vi "HFRR ADV v01.vi"() -> ()   [LabVIEW 2023] (continued)
                  n214 = VISA Read(VISA resource name=w509, byte count=w500, error in (no error)=w508) -> (VISA resource name out=w506:refnum<visa-resource-name>, read buffer=w498:string, error out=w507:errorcluster)  [unwired: 1 out]
                  n215 = Concatenate Strings(w499, w498) -> (w497:string)
                }
                "UnoRead" <- w449
                n216 = while {
                  shift-right: [w483] -> w460
                  shift-left: w449 -> [w489]
                  tunnel: [w482] -> w456 mode=indexing
                  tunnel: [w484] -> _
                  i -> [w484]
                  stop <- w486 stop-if-true
                  n217 = Match Pattern(string=w489, regular expression="*") -> (after substring=w487:string)  [unwired: 1 in, 3 out]
                  n218 = Match Pattern(string=w487, regular expression="&") -> (before substring=w482:string, after substring=w483:string, offset past match=w485:i32)  [unwired: 1 in, 1 out]
                  n219 = Less Than 0?(x=w485) -> (x < 0?=w486:bool)
                }
                n220 = local write "Residual Uno"(w460) -> ()
                n221 = Array Size(array=w456) -> (size(s)=w457:i32)
                n222 = Decrement(x=w457) -> (x-1=w459:i32)
                n223 = Delete From Array(array=w456, length=1, index=w459) -> (array with subset deleted=w454:string[])  [unwired: 1 out]
                n224 = Array Size(array=w454) -> (size(s)=w453:i32)
                n225 = Decrement(x=w453) -> (x-1=w452:i32)
                n226 = while {
                  tunnel: [w481] -> w465 mode=indexing
                  tunnel: [w480] -> w464 mode=indexing
                  tunnel: w454 -> [w474] mode=indexing
                  tunnel: w452 -> [w473]
                  tunnel: [w471] -> _
                  i -> [w471]
                  stop <- w472 stop-if-true
                  w475 = 0 ("length (rest)")
                  w477 = ";" ("regular expression")
                  n227 = Match Pattern(string=w474, regular expression=w477) -> (before substring=w479:string, after substring=w478:string)  [unwired: 1 in, 2 out]
                  n228 = Match Pattern(string=w478, regular expression=w477) -> (before substring=w476:string)  [unwired: 1 in, 3 out]
                  n229 = Less Or Equal?(x=w473, y=w471) -> (x <= y?=w472:bool)
                  n230 = Decimal String To Number(string=w479, default (0L)=w475) -> (number=w481:i32)  [unwired: 1 in, 1 out]
                  n231 = Decimal String To Number(string=w476, default (0L)=w475) -> (number=w480:i32)  [unwired: 1 in, 1 out]
                }
                n232 = Bundle(w465, w464) -> (w455:cluster{i32[], i32[]})  [unwired: 1 in]
                n233 = case shown="0, Default" "ADC Res" {
                  tunnel: [w492 w494] -> w448
                  frame 0, Default {
                    n234 = Divide(x=65535 ("length (rest)"), y=2 ("length (rest)")) -> (x/y=w492:dbl)
                  }
                  frame 1 {
                    n235 = Divide(x=16777216 ("length (rest)"), y=2 ("length (rest)")) -> (x/y=w494:dbl)
                  }
                }
                n236 = Divide(x=w455, y=w448) -> (x/y=w466:cluster{dbl[], dbl[]})
                n237 = Multiply(x=w466, y=sgl 5.03 ("Numeric")) -> (x*y=w463:cluster{dbl[], dbl[]})
                n238 = Unbundle(w463) -> (→"Ch1":dbl[], →"Ch0":dbl[])
              }
            }
          }
          frame #1 {
            n239 = local read "Ch1"() -> (w534:dbl[])
            n240 = call-poly <vilib>:"Mean.vi"("X"=w534) -> ("mean"=w535:dbl)  [unwired: 1 out]
            "Slide 3" <- w535
            n241 = call <vilib>:"Mean PtByPt.vi"("x"=w535, "sample length"=10, "initialize"="Reset 2") -> ("mean"=→"Mean Pos Fil 2":dbl)  [unwired: 1 in, 1 out]
            n242 = case shown="True" "Zero 2" {
              tunnel: w534 -> [_ w564]
              frame False {
              }
              frame True {
                n243 = call-poly <vilib>:"Mean.vi"("X"=w564) -> ("mean"=→"zOff 2":dbl)  [unwired: 1 out]
                n244 = local write "Zero 2"(FALSE ("Zero")) -> ()
              }
            }
            n245 = Tick Count (ms)() -> (millisecond timer value=w551:u32)
            n246 = local read "zOff 2"() -> (w544:dbl)
            n247 = Subtract(x=w551, y=w552) -> (x-y=w550:u32)
            n248 = Subtract(x=w534, y=w544) -> (x-y=w540:dbl[])
            n249 = Divide(x=w550, y=u32 1000 ("x")) -> (x/y=w548:dbl)
            n250 = Multiply(x=w540, y=1.0 ("PG Oth")) -> (x*y=w526:dbl[])
            n251 = Divide(x=w526, y=1) -> (x/y=w525:dbl[])
            "Fric Val" <- w525
            n252 = local read "FF buffer"() -> (w531:dbl[])
            n253 = call-poly <vilib>:"Mean.vi"("X"=w525) -> ("mean"=w539:dbl)  [unwired: 1 out]
            n254 = Array Size(array=w531) -> (size(s)=w533:i32)
            n255 = case shown="True" "DC corr 2" {
              tunnel: w525 -> [w567 w570]
              tunnel: [w567 w569] -> w532
              tunnel: w539 -> [_ w568]
              frame False {
              }
              frame True {
                n256 = Subtract(x=w570, y=w568) -> (x-y=w569:dbl[])
              }
            }
            n257 = Insert Into Array(array=w531, index=w533, new element=w525) -> (w528:dbl[])
            n258 = Array Size(array=w532) -> (size(s)=w547:i32)
            n259 = Array Size(array=w528) -> (size(s)=w527:i32)
            n260 = Divide(x=w547, y=w548) -> (x/y=w543:dbl)
            "Sps 2" <- w543
            n261 = Greater?(x=w527, y=1000) -> (0:w529:bool)
            n262 = Reciprocal(x=w543) -> (1/x=w541:dbl)
            "dt" <- w541
            n263 = case shown="True" w529 {
              tunnel: [w557 w560] -> w516
              tunnel: w528 -> [w557 w563]
              tunnel: w527 -> [_ w562]
              frame False {
              }
              frame True {
                n264 = Subtract(x=w562, y=1000) -> (x-y=w558:i32)
                n265 = Delete From Array(array=w563, length=w558, index=0) -> (array with subset deleted=w560:dbl[])  [unwired: 1 out]
              }
            }
            n266 = Bundle By Name("Y"=w532, "dt"=w541, "t0"=timestamp(0 s since 1904-01-01)) -> (w511:waveform(dbl))  [unwired: 1 in]
            n267 = local read "FRIC. FORCE :"() -> (w513:dbl)
            n268 = call "Elapsed Time5"("Time Target (s)"="check time s", "Reset"="Reset 3") -> ("Time has Elapsed"=w518:bool)  [unwired: 10 in, 7 out]
            n269 = Multiply(x=w513, y=21.1986) -> (x*y=w512:dbl)
            n270 = Multiply(x=w512, y=w511) -> (x*y=→"FF_Wfm":waveform(dbl))
            n271 = Negate(x=w516) -> (-x=w515:dbl[])
            n272 = local write "FF buffer"(w516) -> ()
            n273 = Array Max & Min(array=w515) -> (max value=w523:dbl)  [unwired: 3 out]
            n274 = Greater Or Equal?(x=w523, y="Threshold value") -> (x >= y?=w519:bool)
            n275 = And(x=w519, y=w518) -> (x .and. y?=w517:bool)
            n276 = case shown="True" w517 {
              frame False {
                n277 = local write "Reset 3"(FALSE ("Reset 3")) -> ()
              }
              frame True {
                n278 = local write "save dpt"(TRUE ("save dpt")) -> ()
                n279 = local write "Reset 3"(TRUE ("Reset 3")) -> ()
              }
            }
          }
          frame #2 {
            n280 = local read "FF buffer"() -> (w577:dbl[])
            n281 = Array Max & Min(array=w577) -> (max value=w572:dbl, min value=w573:dbl)  [unwired: 2 out]
            n282 = Multiply(x=1.0 ("y 2"), y="Threshold") -> ()  [unwired: 1 out]
            n283 = Subtract(x=w572, y=w573) -> (x-y=w574:dbl)
            n284 = Greater?(x=w574, y="Threshold") -> (0:w571:bool)
            n285 = case shown="True" w571 {
              tunnel: w577 -> [_ w584]
              tunnel: [_ w582] -> _
              frame False {
              }
              frame True {
                w583 = 1.0 ("y")
                n286 = Delete From Array(array=w584, length=100, index=0) -> (deleted portion=w589:dbl[])  [unwired: 1 out]
                n287 = local read "FRIC. FORCE :"() -> (w582:dbl)
                n288 = call-poly <vilib>:"Mean.vi"("X"=w589) -> ("mean"=w588:dbl)  [unwired: 1 out]
                n289 = Subtract(x=w584, y=w588) -> (x-y=w587:dbl[])
                n290 = Multiply(x=w583, y=w583) -> (x*y=w585:dbl)
                n291 = Multiply(x=w587, y=w585) -> (x*y=w586:dbl[])
                "FF cal val" <- w586
                n292 = Array Max & Min(array=w586) -> (max value=w579:dbl, min value=w578:dbl)  [unwired: 2 out]
                n293 = Array Size(array=w586) -> (size(s)=w580:i32)
                n294 = property on="FF Calibration g" class="WFGraph (strict)"("X Scale.Range:Minimum"=0.0 ("y"), "X Scale.Range:Maximum"=w580, "Y Scale.Range:Minimum"=w579, "Y Scale.Range:Maximum"=w578) -> ()  [unwired: 2 in, 2 out]
              }
            }
          }
          frame #3 {
            # "5"
            n295 = local read "Ch0"() -> (w606:dbl[])
            n296 = local read "DISPLACEMENT :"() -> (w677:dbl)
            n297 = local read "zOff 3"() -> (w680:dbl)
            n298 = Add(x=w606, y="Offset") -> (x+y=w605:dbl[])
            n299 = Subtract(x=w606, y=w680) -> (x-y=w663:dbl[])
            n300 = Multiply(x=w677, y=1.0) -> (x*y=w593:dbl)
            n301 = Multiply(x=w605, y="Gain") -> (x*y=w600:dbl[])
            "Voltage LVDT Acq" <- w600
            "gLVDTraw" <- w600
            n302 = case shown="True" "Zero 3" {
              tunnel: w606 -> [_ w695]
              frame False {
              }
              frame True {
                n303 = call-poly <vilib>:"Mean.vi"("X"=w695) -> ("mean"=→"zOff 3":dbl)  [unwired: 1 out]
                n304 = local write "Zero 3"(FALSE ("Zero")) -> ()
              }
            }
            n305 = Multiply(x=w593, y="DISPLACEMENT : 2") -> (x*y=w660:dbl)
            n306 = call-poly <vilib>:"Mean.vi"("X"=w600) -> ("mean"=w599:dbl)  [unwired: 1 out]
            n307 = Array Max & Min(array=w600) -> (max value=w604:dbl, min value=w603:dbl)  [unwired: 2 out]
            n308 = Multiply(x=w663, y=w593) -> (x*y=w676:dbl[])
            "ABS DP" <- w676
            n309 = Multiply(x=w663, y=w660) -> (x*y=w662:dbl[])
            n310 = local read "Standard Slip Gauge (mm)"() -> (w661:dbl)
            n311 = Subtract(x=w604, y=w603) -> (x-y=→"Pk-Pk":dbl)
            n312 = call-poly <vilib>:"Mean.vi"("X"=w676) -> ("mean"=w665:dbl)  [unwired: 1 out]
            n313 = call-poly <vilib>:"Mean.vi"("X"=w662) -> ("mean"=w592:dbl)  [unwired: 1 out]
            "Disp (mm)" <- w592
            "software msrnt" <- w592
            n314 = Subtract(x=w599, y="LvdtOff") -> (x-y=w598:dbl)
            n315 = case shown="True" "DC correction" {
              tunnel: w676 -> [w698 w701]
              tunnel: [w698 w700] -> w612
              tunnel: w665 -> [_ w699]
              frame False {
              }
              frame True {
                n316 = Subtract(x=w701, y=w699) -> (x-y=w700:dbl[])
              }
            }
            n317 = Threshold 1D Array(2:0.0 ("threshold y"), 3:w612) -> (0:w629:dbl)  [unwired: 1 in]
            n318 = Divide(x=w592, y=w661) -> (x/y=w659:dbl)
            n319 = Multiply(x=w659, y=w660) -> (x*y=→"DISPLACEMENT : 3":dbl)
            n320 = Equal To 0?(x=w629) -> (x = 0?=w630:bool)
            n321 = local read "dt"() -> (w679:dbl)
            n322 = case shown="True" w630 {
              tunnel: w612 -> [_ w689]
              tunnel: [w685 w686] -> w625
              tunnel: w629 -> [w685 _]
              frame False {
              }
              frame True {
                n323 = Threshold 1D Array(1:20 ("start index (0)"), 2:0.0 ("threshold y"), 3:w689) -> (0:w686:dbl)
              }
            }
            n324 = Bundle By Name("Y"=w612, "dt"=w679, "t0"=timestamp(0 s since 1904-01-01)) -> (w667:waveform(dbl))  [unwired: 1 in]
            n325 = local read "FF_Wfm"() -> (w666:waveform(dbl))
            n326 = call-poly <vilib>:"Extract Single Tone Information.vi"("time signal in"=w667) -> ("detected amplitude"=w601:dbl, "detected frequency"=→"Freq":dbl)  [unwired: 5 in, 4 out]
            n327 = Subtract(x=w598, y=w601) -> (x-y=w610:dbl)
            n328 = Add(x=w601, y=w598) -> (x+y=w609:dbl)
            n329 = Bundle(w598, w610, w609) -> (→"Slide 8":cluster{dbl, dbl, dbl})  [unwired: 1 in]
            n330 = Build Array(w667, w666) -> (w648:waveform(dbl)[])
            "Waveform Graph 2" <- w648
            n331 = Split 1D Array(array=w612, index=w625) -> (second subarray=w626:dbl[])  [unwired: 1 out]
            n332 = Index Array(array=w648) -> (element #1=w649:waveform(dbl), element #2=w651:waveform(dbl))  [unwired: 2 in]
            n333 = Multiply(x=w601, y=2.0) -> (x*y=w668:dbl)
            "Stroke" <- w668
            "Mean(RAW) Stroke" <- w668
            n334 = local read "Test \nStatus"() -> (w669:bool)
            n335 = Threshold 1D Array(1:180 ("start index (0)"), 2:0.0 ("threshold y"), 3:w626) -> (0:w624:dbl)
            n336 = Unbundle By Name(w649) -> ("Y"=w622:dbl[])
            n337 = Unbundle By Name(w651) -> ("Y"=w623:dbl[])
            n338 = Split 1D Array(array=w623, index=w625) -> (second subarray=w620:dbl[])  [unwired: 1 out]
            n339 = In Range and Coerce(upper limit=1.5, x=w668, lower limit=0.5) -> (In Range?=w672:bool)  [unwired: 1 out]
            n340 = Split 1D Array(array=w626, index=w624) -> (first subarray=w619:dbl[])  [unwired: 1 out]
            n341 = Split 1D Array(array=w620, index=w624) -> (first subarray=w617:dbl[])  [unwired: 1 out]
            n342 = Split 1D Array(array=w622, index="Window") -> (second subarray=w640:dbl[])  [unwired: 1 out]
            n343 = Not(x=w672) -> (.not. x?=w671:bool)
            n344 = And(x=w671, y=w669) -> (x .and. y?=w670:bool)
            n345 = case shown="True" w670 {
              tunnel: [i32[] [] w691] -> _
              frame False {
              }
              frame True {
                n346 = local read "Array"() -> (w694:string[])
                n347 = local read "UnoRead"() -> (w693:string)
                n348 = Build Array (concatenate)(w694, w693) -> (w692:string[])
                "Array" <- w692
                n349 = String Length(string=w692) -> (length=w691:i32[])
              }
            }
            n350 = Array Max & Min(array=w623) -> (max value=w652:dbl, min value=w653:dbl)  [unwired: 2 out]
            n351 = Array Max & Min(array=w640) -> (max value=w654:dbl, min value=w655:dbl)  [unwired: 2 out]
            n352 = call-poly <vilib>:"Hanning Window.vi"("X"=w619) -> ("Windowed X"=w618:dbl[])  [unwired: 1 out]
            n353 = call-poly <vilib>:"Hanning Window.vi"("X"=w617) -> ("Windowed X"=w616:dbl[])  [unwired: 1 out]
            n354 = Subtract(x=w654, y=w655) -> (x-y=w656:dbl)
            n355 = Subtract(x=w652, y=w653) -> (x-y=w657:dbl)
            n356 = Build Array(w618, w616) -> (→"Waveform Graph 4":dbl[][])
            n357 = local read "G_val"() -> (w642:dbl)
            n358 = Divide(x=w657, y=w656) -> (x/y=w645:dbl)
            n359 = call-poly <vilib>:"RMS.vi"("X"=w640) -> ("rms value"=w596:dbl)  [unwired: 1 out]
            "Current (A)" <- w596
            n360 = call-poly <vilib>:"RMS.vi"("X"=w617) -> ("rms value"=w641:dbl)  [unwired: 1 out]
            n361 = local read "Constant (G)"() -> (w634:dbl)
            n362 = Multiply(x=w645, y=0.2) -> (x*y=w647:dbl)
            n363 = Multiply(x=0.8 ("y"), y=w642) -> (x*y=w646:dbl)
            n364 = Divide(x=w641, y=w596) -> (x/y=w635:dbl)
            n365 = Add(x=w647, y=w646) -> (x+y=w614:dbl)
            n366 = Not A Number/Path/Refnum?(number/path/refnum=w614) -> (NaN/Path/Refnum?=w613:bool)
            n367 = Multiply(x=w635, y=0.2) -> (x*y=w636:dbl)
            n368 = Multiply(x=0.8 ("y"), y=w634) -> (x*y=w637:dbl)
            n369 = Select(t=0.0, s=w613, f=w614) -> (s? t:f=w594:dbl)
            "G_val" <- w594
            n370 = Multiply(x=w596, y=w594) -> (x*y=→"Friction Force (N)":dbl)
            n371 = Add(x=w636, y=w637) -> (x+y=w633:dbl)
            "Constant (G)" <- w633
            n372 = Bundle(w633, "t"=w594) -> (→"pk-pk":cluster{dbl, "t":dbl})  [unwired: 1 in]
          }
          frame #4 {
            # "C:\\WinDucom\\data\\"
            # "?C:\\LAB-IQ-NXT\\data"
            n373 = case shown="True" "save dpt" {
              frame False {
              }
              frame True {
                n374 = local read "FF buffer"() -> (w713:dbl[])
                n375 = local read "ABS DP"() -> (w712:dbl[])
                n376 = Build Array(w713, w712) -> (w708:dbl[][])
                n377 = Transpose 2D Array(2D array=w708) -> (transposed array=w707:dbl[][])
                n378 = Array To Spreadsheet String(delimiter (Tab)=";", array=w707, 3:"" ("format string")) -> (spreadsheet string=w709:string)
                "String 9" <- w709
                n379 = Concatenate Strings("FF ( V ); DP( mincron ) " ("character string"), "\r") -> (w722:string)
                n380 = local read "file count"() -> (w705:i32)
                n381 = local read "FILE 2"() -> (w710:string)
                n382 = local write "save dpt"(FALSE ("Hold 3")) -> ()
                n383 = Number To Decimal String(number=w705) -> (decimal integer string=w711:string)  [unwired: 1 in]
                n384 = Concatenate Strings(w710, w711) -> (w703:string)
                n385 = Concatenate Strings("C:\\LAB-IQ-NXT\\data" ("Substring"), w703) -> (w718:string)
                n386 = Concatenate Strings(w718, ".dpf" ("Substring")) -> (w716:string)
                n387 = Add(x=1, y=w705) -> (x+y=w706:i32)
                n388 = local write "file count"(w706) -> ()
                n389 = String To Path(string=w716) -> (path=w714:path)
                n390 = call <vilib>:"Write Characters To File.vi"("append to file? (new file:F)"=FALSE, "character string"=w722, "file path (dialog if empty)"=w714) -> ("new file path (Not A Path if cancelled)"=w719:path)  [unwired: 2 in]
                n391 = call <vilib>:"Write Characters To File.vi"("append to file? (new file:F)"=TRUE, "character string"=w709, "file path (dialog if empty)"=w719) -> ()  [unwired: 2 in, 1 out]
              }
            }
          }
          frame #5 {
            n392 = case shown="True" "Hold 4" {
              frame False {
              }
              frame True {
                n393 = File Dialog(6:"*.dpf" ("pattern"), 11:path "C:/LAB-IQ-NXT" ("start path")) -> (0:w729:errorcluster, 3:w744:path)  [unwired: 5 in, 2 out]
                n394 = Unbundle(w729) -> ()  [unwired: 3 out]
                n395 = call <vilib>:"Read Characters From File.vi"("file path (dialog if empty)"=w744) -> ("character string"=w734:string)  [unwired: 5 in, 3 out]
                n396 = Spreadsheet String To Array(delimiter (Tab)=";", format string="%S", spreadsheet string=w734, array type (2D Dbl)=string[][] []) -> (array=w738:string[][])
                n397 = for {
                  tunnel: w738 -> [w748] mode=indexing
                  tunnel: [w747] -> w739 mode=indexing
                  n398 = for {
                    tunnel: w748 -> [w750] mode=indexing
                    tunnel: [w749] -> w747 mode=indexing
                    n399 = call <vilib>:"Trim Whitespace.vi"("string"=w750) -> ("trimmed string"=w749:string)  [unwired: 1 in]
                  }
                }
                n400 = Fract/Exp String To Number(string=w739) -> (number=w741:dbl[][])  [unwired: 3 in, 1 out]
                n401 = Array Subset(array=w741, index (row)=1 ("index (col)")) -> (w743:dbl[][])  [unwired: 3 in]
                n402 = Index Array(array=w743, index (col) #1=0 ("disabled index (col)"), index (col) #2=1 ("disabled index (col)")) -> (element #1=w732:dbl[], element #2=w731:dbl[])  [unwired: 2 in]
                n403 = Build Array(w732, w731) -> (→"Waveform Graph":dbl[][])
              }
            }
          }
        }
      }
      frame Error {
        w766 = u16 0 items=["None", "XON/XOFF", "RTS/CTS", "XON/XOFF & RTS/CTS", "DTR/DSR", "XON/XOFF & DTR/DSR"] ("flow control (0:none)  2")
        w764 = u16 10 items=["1.0"=10, "1.5"=15, "2.0"=20] ("stop bits 2")
        w762 = u16 0 items=["None", "Odd", "Even", "Mark", "Space"] ("parity 2")
        w763 = u32 10000  # timeout (10sec)
        n404 = VISA Close(VISA resource name=w758, error in (no error)=w755) -> (error out=w759:errorcluster)
        n405 = local read "Com Port 1"() -> (w751:refnum<visa-resource-name>)
        n406 = call <vilib>:"Clear Errors.vi"("error in (no error)"=w759) -> ("error out"=w756:errorcluster)  [unwired: 5 in, 1 out]
        n407 = local write "Sps 3"(0.0 ("Sps 4")) -> ()
        n408 = call-poly "VISA Configure Serial Port"("VISA resource name"=w751, "timeout (10sec)"=w763, "baud rate (9600)"=u32 250000 ("baud rate  2"), "data bits (8)"=u16 8 ("data bits  2"), "parity (0:none)"=w762, "error in (no error)"=w756, "stop bits (10: 1 bit)"=w764, "flow control (0:none)"=w766) -> ("VISA resource name out"=w767:refnum<visa-resource-name>, "error out"=w768:errorcluster)  [unwired: 6 in]
        n409 = flat-sequence {
          tunnel: w767 -> [w770]
          tunnel: w768 -> [w769]
          tunnel: [w770] -> w760
          tunnel: [w769] -> w752
          frame #0 {
            n410 = Wait (ms)(milliseconds to wait=u32 50) -> ()  [unwired: 1 out]
          }
        }
        "Residual Uno" <- ""
        "Port 1 Error" <- w752
      }
    }
    n411 = local read "Port 1a"() -> (w413:bool)
    n412 = local read "Port 3"() -> (w414:bool)
    n413 = Or(x=w414, y=w413) -> (x .or. y?=w416:bool)
    n414 = case shown="False" w416 {
      frame False {
        w427 = FALSE ("Visible")
        n415 = property on="Port 1a" class="Bool (strict)"("Visible"=w427) -> ()  [unwired: 2 in, 2 out]
        n416 = property on="Port 3" class="Bool (strict)"("Visible"=w427) -> ()  [unwired: 2 in, 2 out]
      }
      frame True {
        w428 = TRUE ("Visible")
        n417 = property on="Port 1a" class="Bool (strict)"("Visible"=w428) -> ()  [unwired: 2 in, 2 out]
        n418 = property on="Port 3" class="Bool (strict)"("Visible"=w428) -> ()  [unwired: 2 in, 2 out]
      }
    }
    n419 = local read "EXIT"() -> (w418:bool)
    "Error Uno" <- w412
  }
  n420 = while {
    tunnel: w47 -> [_]
    tunnel: [w801] -> _
    tunnel: w16 -> [_]
    tunnel: ["EXIT"] -> w44
    i -> [w801]
    stop <- "EXIT" stop-if-true
    # "C:\\LAB-IQ-NXT\\Scar View.exe"
    n421 = local read "RUN"() -> (w799:bool)
    n422 = local read "EDIT 2"() -> (w786:bool)
    n423 = case shown="False" w799 {
      frame False {
        n424 = local read "stopT"() -> (w1691:bool)
        n425 = case shown="True" w1691 {
          frame False {
          }
          frame True {
            w1692 = FALSE
            n426 = local write "st enable"(w1692) -> ()
            n427 = local write "stopT"(w1692) -> ()
          }
        }
      }
      frame True {
        "stopT" <- TRUE
      }
    }
    n428 = case shown="True" "EDIT 3" {
      frame False {
      }
      frame True {
        n429 = local write "EDIT 3"(FALSE ("EDIT 3")) -> ()
        n430 = local write "Main Tab"(T1."About" ("Main Tab")) -> ()
      }
    }
    n431 = case shown="True" w786 {
      frame False {
        n432 = local write "Password 2"("" ("Password")) -> ()
        n433 = property on="Password 2" class="Str"("Visible"=FALSE) -> ()  [unwired: 2 in, 2 out]
      }
      frame True {
        n434 = property on="Password 2" class="Str"("Visible"=TRUE) -> ()  [unwired: 2 in, 2 out]
        n435 = Equal?(x="Password 2", y="HFRR1234") -> (x = y?=w831:bool)
        n436 = case shown="True" w831 {
          tunnel: "Password 2" -> [w834 _]
          frame False {
            n437 = String Length(string=w834) -> (length=w835:i32)
            n438 = Greater Than 0?(x=w835) -> (x > 0?=w833:bool)
            n439 = case shown="False" w833 {
              frame False {
                n440 = property on="Password 2" class="Str"("Caption.Text"="Password (Advance Setting)") -> ()  [unwired: 2 in, 2 out]
              }
              frame True {
                n441 = property on="Password 2" class="Str"("Caption.Text"="Incorrect Password!") -> ()  [unwired: 2 in, 2 out]
              }
            }
          }
          frame True {
            n442 = local write "Password 2"("" ("Password")) -> ()
            n443 = local write "Main Tab"(T1."Advance" ("Main Tab")) -> ()
            n444 = local write "EDIT 2"(FALSE ("EDIT 2")) -> ()
          }
        }
      }
    }
    n445 = Wait (ms)(milliseconds to wait=u32 50) -> ()  [unwired: 1 out]
    n446 = local read "EXIT 2"() -> (w779:bool)
    n447 = local read "Configure"() -> (w782:bool)
    n448 = local read "Analysis"() -> (w781:bool)
    n449 = local read "Home 9"() -> (w776:bool)
    n450 = local read "Home"() -> (w775:bool)
    n451 = local read "STOP 2"() -> (w778:bool)
    n452 = local read "Home 8"() -> (w777:bool)
    n453 = local read "Re-Initialise"() -> (w784:bool)
    n454 = case shown="True" w779 {
      selector: w779 -> [_ w812]
      frame False {
      }
      frame True {
        n455 = local write "EXIT"(w812) -> ()
        n456 = local write "EXIT 2"(FALSE ("EXIT 2")) -> ()
        n457 = local write "Main Tab"(T1."HOME" ("Main Tab")) -> ()
      }
    }
    n458 = case shown="True" w775 {
      frame False {
      }
      frame True {
        n459 = local write "Home"(FALSE ("Home")) -> ()
        n460 = local write "Main Tab"(T1."HOME" ("Main Tab")) -> ()
      }
    }
    n461 = case shown="True" w784 {
      frame False {
      }
      frame True {
        n462 = local write "Re-Initialise"(FALSE ("Re-Initialise")) -> ()
      }
    }
    n463 = case shown="True" w776 {
      frame False {
      }
      frame True {
        n464 = local write "Main Tab"(T1."HOME" ("Main Tab")) -> ()
        n465 = local write "Home 9"(FALSE ("Home 9")) -> ()
      }
    }
    n466 = case shown="True" w777 {
      frame False {
      }
      frame True {
        n467 = local write "Home 8"(FALSE ("Home 8")) -> ()
        n468 = local write "Main Tab"(T1."HOME" ("Main Tab")) -> ()
      }
    }
    n469 = case shown="True" w778 {
      frame False {
      }
      frame True {
        n470 = local write "STOP 2"(FALSE ("STOP 2")) -> ()
        n471 = local write "Main Tab"(T1."HOME" ("Main Tab")) -> ()
      }
    }
    n472 = case shown="True" w782 {
      frame False {
      }
      frame True {
        n473 = local write "Configure"(FALSE) -> ()
        n474 = local write "Main Tab"(T1."Acquire" ("Main Tab")) -> ()
      }
    }
    n475 = local read "service 2"() -> (w780:bool)
    n476 = case shown="True" w781 {
      frame False {
      }
      frame True {
        n477 = local write "Analysis"(FALSE) -> ()
        n478 = local write "Main Tab"(T1."Compare Files" ("Main Tab")) -> ()
      }
    }
    n479 = case shown="\"ASTM D6079\", Default" "TEST STANDARD" {
      tunnel: [2.0 ("Set Temp") 0.0 ("Set Temp") 2.0 ("Set Temp") 0.0 ("Set Temp")] -> w787
      frame "ASTM D6079", Default {
        # "astm hide"
        n480 = local write "Set Hz"(50.0 ("Hz")) -> ()
        n481 = local write "Set Strk"(1.0 ("Set Strk")) -> ()
        n482 = local write "Set Rh"(53.0 ("Set Rh")) -> ()
        n483 = local write "Set Temp"(60.0 ("Set Temp")) -> ()
        n484 = local write "test time"(75.0 ("test time")) -> ()
        n485 = local write "NORMAL LOAD"(2.0 ("NORMAL LOAD")) -> ()
        "Test Standard" <- "ASTM D6079" ("Test Standard 2")
      }
      frame "ISO 12156" {
        n486 = local write "Set Hz"(50.0 ("Hz")) -> ()
        n487 = local write "Set Rh"(53.0 ("Set Rh")) -> ()
        n488 = local write "Set Strk"(1.0 ("Set Strk")) -> ()
        n489 = local write "test time"(75.0 ("test time")) -> ()
        n490 = local write "Set Temp"(60.0 ("Set Temp")) -> ()
        n491 = local write "NORMAL LOAD"(2.0 ("NORMAL LOAD")) -> ()
      }
      frame "CEC F-096-A-06" {
        n492 = local write "Set Strk"(1.0 ("Set Strk")) -> ()
        n493 = local write "Set Hz"(50.0 ("Hz")) -> ()
        n494 = local write "Set Rh"(53.0 ("Set Rh")) -> ()
        n495 = local write "Set Temp"(60.0 ("Set Temp")) -> ()
        n496 = local write "test time"(75.0 ("test time")) -> ()
        n497 = local write "NORMAL LOAD"(2.0 ("NORMAL LOAD")) -> ()
      }
      frame "Custom" {
      }
    }
    n498 = local read "OPEN 6"() -> (w783:bool)
    n499 = local read "service 3"() -> (w773:bool)
    n500 = case shown="True" w780 {
      frame False {
      }
      frame True {
        n501 = local write "service 2"(FALSE) -> ()
        n502 = local write "Main Tab"(T1."About" ("Main Tab")) -> ()
      }
    }
    n503 = Or(x=w783, y=w773) -> (x .or. y?=w774:bool)
    n504 = local read "RUN"() -> (w796:bool)
    n505 = case shown="True" w774 {
      selector: w774 -> [_ w823]
      frame False {
      }
      frame True {
        n506 = Not(x=w823) -> (.not. x?=w819:bool)
        n507 = local write "service 3"(w819) -> ()
        n508 = local write "OPEN 6"(w819) -> ()
        n509 = call <vilib>:"System Exec.vi"("wait until completion? (T)"=TRUE, "command line"="C:\\LAB-IQ-NXT\\Scar View.exe") -> ("error out"=→"error out 5":errorcluster)  [unwired: 6 in, 3 out]
      }
    }
    n510 = case shown="True" w796 {
      frame False {
      }
      frame True {
        n511 = local read "Main Tab"() -> (w1689:T1)
        n512 = case shown="\"Compare Files\"" w1689 {
          frame "Acquire", Default {
          }
          frame "Compare Files" {
            n513 = local write "Main Tab"(T1."Acquire" ("Main Tab")) -> ()
          }
          frame "About" {
          }
        }
      }
    }
    n514 = local read "Main Tab"() -> (w772:T1)
    n515 = case shown="\"Acquire\", Default" w772 {
      tunnel: [T1."Acquire" ("Main Tab") T10."   COMPARE   FILES " ("Tab Control") T11."PRINT REPORT" ("Tab Control")] -> w794
      frame "Acquire", Default {
      }
      frame "Compare Files" {
      }
      frame "About" {
      }
    }
    n516 = property on="SetTemp" class="DigNum (strict)"("Disabled"=w787) -> ()  [unwired: 2 in, 2 out]
    n517 = case shown="0, Default" w794 {
      frame 0, Default {
        w1833 = 0.2 ("y")
        w1838 = 1.0 ("y")
        w1839 = 0.8 ("y")
        # "Elapsed time\ncof\nstroke\nAir temp\nTemp\nHumidity"
        n518 = case shown="True" "Save & Continue" {
          frame False {
          }
          frame True {
            "acq 2" <- TRUE ("acq 2")
          }
        }
        n519 = case shown="True" "Save & Continue" {
          frame False {
          }
          frame True {
            n520 = while {
              tunnel: "0123456789abcdefghijklmnopqrstuvwxyzABCDEFGHIJKLMNOPQRSTUVWXYZ" ("string 2") -> [w1957]
              shift-right: [w1955] -> w1950
              shift-left: "" -> [w1954]
              i -> [w1964]
              stop <- w1963 stop-if-true
              n521 = Random Number (0-1)() -> (number: 0 to 1=w1958:dbl)
              n522 = Multiply(x=w1958, y=62.0) -> (x*y=w1960:dbl)
              n523 = Decrement(x="Length") -> (x-1=w1953:i16)
              n524 = To Word Integer(number=w1960) -> (16bit integer=w1961:i16)
              n525 = String Subset(string=w1957, offset (0)=w1961, length (rest)=1 ("length (rest)")) -> (substring=w1956:string)
              n526 = Greater Or Equal?(x=w1964, y=w1953) -> (x >= y?=w1963:bool)
              n527 = Concatenate Strings(w1956, w1954) -> (w1955:string)
            }
            n528 = local write "UUID"(w1950) -> ()
          }
        }
        n529 = case shown="True" "Save & Continue" {
          frame False {
          }
          frame True {
            n530 = local read "Operator ID"() -> (w2240:string)
            n531 = local read "FILE"() -> (w2247:string)
            n532 = String Length(string=w2240) -> (length=w2241:i32)
            n533 = String Length(string=w2247) -> (length=w2245:i32)
            n534 = Greater?(x=w2241, y=0) -> (0:w2239:bool)
            n535 = Greater?(x=w2245, y=0) -> (0:w2244:bool)
            n536 = And(x=w2244, y=w2239) -> (x .and. y?=w2243:bool)
            n537 = case shown="True" w2243 {
              frame False {
                n538 = stacked-sequence {
                  frame #0 {
                    n539 = One Button Dialog(message="Please Enter a File Name and Operator ID to save data !", button name ("OK")="Ok") -> ()  [unwired: 1 out]
                  }
                  frame #1 {
                    n540 = local write "Save & Continue"(FALSE ("OK Button")) -> ()
                  }
                }
                n541 = local write "Save & Continue"(FALSE ("OK Button")) -> ()
              }
              frame True {
                n542 = stacked-sequence {
                  frame #0 {
                    (unwired) ")!" ("string")
                    (unwired) ")" ("string")
                    w2252 = dbl[] [] ("History Data")
                    w2256 = "\r"
                    # "C:\\WinDucom\\Data\\"
                    # "C:\\LAB-IQ-NXT\\data"
                    n543 = local read "Batch Ref Num :"() -> (w2254:string)
                    n544 = local read "NORMAL LOAD"() -> (w2273:dbl)
                    n545 = local read "Fuel Discription :"() -> (w2267:string)
                    n546 = Multiply(x=w2273, y=1.0) -> (x*y=w2272:dbl)
                    n547 = Number To Fractional String(number=w2272, width (-)=i16 5, precision (6)=i16 2) -> (F-format string=w2281:string)  [unwired: 1 in]
                    n548 = Concatenate Strings(w2267) -> (w2268:string)
                    n549 = local read "Remarks :"() -> (w2266:string)
                    n550 = property on="Electronic contact resistance ( % )" class="WFChart (strict)"("History Data"=w2252) -> ()  [unwired: 2 in, 2 out]
                    n551 = Get Date/Time String(date format (0)=enum16{"short", "long", "abbreviated"}."short") -> (date string=w2292:string, time string=w2289:string)  [unwired: 2 in]
                    n552 = property on="Coefficient of Friction" class="WFChart (strict)"("History Data"=w2252) -> ()  [unwired: 2 in, 2 out]
                    n553 = property on="Frictional Force ( N )" class="WFChart (strict)"("History Data"=w2252) -> ()  [unwired: 2 in, 2 out]
                    n554 = Concatenate Strings(w2254) -> (w2253:string)
                    n555 = Concatenate Strings(w2266, "," ("string")) -> (w2265:string)
                    n556 = Concatenate Strings("Load :- " ("Substring"), w2281, " N ," ("Substring")) -> (w2280:string)
                    n557 = local read "String 41"() -> (w2258:string)
                    n558 = local read "FILE"() -> (w2300:string)
                    n559 = Concatenate Strings("(" ("Substring"), w2292, ")" ("Substring"), w2289) -> (w2260:string)
                    "concatenated string" <- w2260
                    n560 = Concatenate Strings("C:\\LAB-IQ-NXT\\data\\" ("string"), w2300) -> (w2299:string)
                    n561 = Concatenate Strings("tested by") -> (w2262:string)
                    n562 = Concatenate Strings(w2299, ".duf" ("Substring")) -> (w2296:string)
                    n563 = Concatenate Strings(w2299, ".dgf" ("Substring")) -> (w2295:string)
                    n564 = String To Path(string=w2295) -> (path=w2293:path)
                    n565 = String To Path(string=w2296) -> (path=w2270:path)
                    n566 = Concatenate Strings(w2258, w2256, "Fuel Discription :-" ("Substring"), w2268, w2256, w2280, w2256, "Batch Ref Num :-" ("Substring"), w2253, w2256, " Remarks :- " ("Substring"), w2265, w2256, " Date :- " ("Substring"), w2260, w2256, "Tested By :-" ("Substring"), w2262) -> (w2274:string)
                    "REMARKS" <- w2274
                    n567 = local write "clk"(0.0 ("clk")) -> ()
                    n568 = local write "speedop"(0.0 ("PIDclk 2")) -> ()
                    n569 = Concatenate Strings("  TIME;      COF;       STROKE;     AIR TEMP;  TEMP;  HUMIDITY;  ECR; PID-OUT; FREQUENCY" ("Substring"), "\r") -> (w2276:string)
                    n570 = call <vilib>:"Write Characters To File.vi"("append to file? (new file:F)"=FALSE, "character string"=w2276, "file path (dialog if empty)"=w2293) -> ()  [unwired: 2 in, 1 out]
                    n571 = call <vilib>:"Write Characters To File.vi"("append to file? (new file:F)"=FALSE, "character string"=w2274, "file path (dialog if empty)"=w2270) -> ()  [unwired: 2 in, 1 out]
                  }
                  frame #1 {
                    n572 = local write "autostrtflg"(TRUE ("autostrtflg")) -> ()
                    n573 = local write "Save & Continue"(FALSE ("OK")) -> ()
                    n574 = local write "STOP 3"(FALSE ("STOP")) -> ()
                    n575 = One Button Dialog(message="Please ensure sample is mounted properly and machine is ready in all aspects for testing !", button name ("OK")="Ok") -> ()  [unwired: 1 out]
                    n576 = property on="Save & Continue" class="Bool (strict)"("Visible"=FALSE ("OK")) -> ()  [unwired: 2 in, 2 out]
                    n577 = property on="STOP 3" class="Bool (strict)"("Visible"=TRUE) -> ()  [unwired: 2 in, 2 out]
                    n578 = Get Date/Time In Seconds() -> (seconds since 1Jan1904=w2305:timestamp)
                    n579 = local write "Cycles elapsed"(0 ("Cycles elapsed")) -> ()
                    n580 = To Double Precision Float(number=w2305) -> (double precision float=w2304:dbl)
                    n581 = local write "cyclecount"(0 ("cyclecount")) -> ()
                    n582 = local write "acq timer"(w2304) -> ()
                    n583 = local write "Save"(FALSE ("Save")) -> ()
                  }
                }
              }
            }
          }
        }
        n584 = case shown="True" "Case Constant\n(See Context Help) 15" {
          frame False {
          }
          frame True {
            n585 = local read "zflag 2"() -> (w1865:dbl)
            n586 = local read "yflag"() -> (w1867:dbl)
            n587 = Equal?(x=w1865, y=3.0 ("tflag")) -> (x = y?=w1868:bool)
            n588 = Equal?(x=w1867, y=2.0 ("tflag")) -> (x = y?=w1869:bool)
            n589 = And(x=w1869, y=w1868) -> (x .and. y?=w1863:bool)
            n590 = case shown="True" w1863 {
              frame False {
              }
              frame True {
                w1894 = 0.0 ("zflag")
                n591 = local read "SEN.RUN HRS"() -> (w1880:dbl)
                n592 = local read "SENSOR TIME"() -> (w1878:dbl)
                n593 = local read "Total No. of Tests"() -> (w1881:dbl)
                n594 = Delete(path (use dialog)=path "C:/LAB-IQ-NXT/WO 2449 TRH.sig" ("file path (dialog if empty)")) -> (deleted path=w1888:path)  [unwired: 4 in, 2 out]
                n595 = Add(x=w1878, y=w1880) -> (x+y=w1879:dbl)
                "SEN.RUN HRS" <- w1879
                n596 = Number To Decimal String(number=w1879) -> (decimal integer string=w1885:string)  [unwired: 1 in]
                n597 = call <vilib>:"compatOverwrite.vi"("overwrite (F)"=TRUE) -> ("overwrite?"=w1874:T14)
                n598 = Delete(path (use dialog)=path "C:/LAB-IQ-NXT/WO 2449 TT.sig" ("file path (dialog if empty)")) -> (deleted path=w1893:path)  [unwired: 4 in, 2 out]
                n599 = Open/Create/Replace File(file path (use dialog)=w1888, operation (0:open)=w1874) -> (refnum out=w1875:refnum<file>, error out=w1876:errorcluster)  [unwired: 4 in, 1 out]
                n600 = Number To Decimal String(number=w1881) -> (decimal integer string=w1889:string)  [unwired: 1 in]
                n601 = Deny Access(4:w1876, 6:T12."deny none" ("deny mode (2)"), 7:w1875) -> (3:w1884:refnum<file>)  [unwired: 1 out]
                n602 = call <vilib>:"compatOverwrite.vi"("overwrite (F)"=TRUE) -> ("overwrite?"=w1870:T14)
                n603 = Write to Binary File(file (use dialog)=w1884, data=w1885, 5:FALSE ("prepend array or string size? (T)")) -> ()  [unwired: 3 in, 3 out]
                n604 = Open/Create/Replace File(file path (use dialog)=w1893, operation (0:open)=w1870) -> (refnum out=w1871:refnum<file>, error out=w1872:errorcluster)  [unwired: 4 in, 1 out]
                n605 = Deny Access(4:w1872, 6:T12."deny none" ("deny mode (2)"), 7:w1871) -> (3:w1892:refnum<file>)  [unwired: 1 out]
                n606 = local write "zflag"(w1894) -> ()
                n607 = local write "zflag 2"(w1894) -> ()
                n608 = Write to Binary File(file (use dialog)=w1892, data=w1889, 5:FALSE ("prepend array or string size? (T)")) -> ()  [unwired: 3 in, 3 out]
              }
            }
          }
        }
        n609 = case shown="True" "STOP 3" {
          frame False {
          }
          frame True {
            w2232 = "" ("Sample ID :")
            (unwired) FALSE ("Visible")
            n610 = local write "Save & Continue"(FALSE ("OK Button")) -> ()
            n611 = local write "STOP 3"(FALSE ("STOP")) -> ()
            n612 = local write "clk"(0.0 ("clk")) -> ()
            n613 = local write "RUN"(FALSE ("OK Button 2")) -> ()
            n614 = property on="Save & Continue" class="Bool (strict)"("Visible"=TRUE) -> ()  [unwired: 2 in, 2 out]
            n615 = property on="STOP 3" class="Bool (strict)"("Visible"=FALSE) -> ()  [unwired: 2 in, 2 out]
            n616 = property on="STOP 2" class="Bool (strict)"("Disabled"=u8 0) -> ()  [unwired: 2 in, 2 out]
            n617 = local write "Fuel Discription :"(w2232) -> ()
            n618 = local write "Remarks :"(w2232) -> ()
            n619 = local write "tested by"(w2232) -> ()
            n620 = local write "FILE"(w2232) -> ()
            n621 = local write "Batch Ref Num :"(w2232) -> ()
          }
        }
        n622 = local read "AIR TEMP"() -> (w1805:dbl)
        n623 = local read "run replace"() -> (w1845:bool)
        n624 = Greater Or Equal?(x=w1805, y=15.0) -> (x >= y?=w1806:bool)
        "powstat" <- w1806
        n625 = local read "acq 2"() -> (w1844:bool)
        n626 = And(x=w1844, y=w1845) -> (x .and. y?=w1843:bool)
        n627 = local read "run replace"() -> (w1846:bool)
        n628 = case shown="True" w1843 {
          frame False {
            n629 = local write "tfalg"(0.0 ("tfalg")) -> ()
          }
          frame True {
            n630 = local read "tfalg"() -> (w1941:dbl)
            n631 = Equal?(x=w1941, y=0.0) -> (x = y?=w1942:bool)
            n632 = case shown="True" w1942 {
              frame False {
              }
              frame True {
                n633 = local read "Total No. of Tests"() -> (w1945:dbl)
                n634 = Increment(x=w1945) -> (x+1=w1944:dbl)
                n635 = local write "Total No. of Tests"(w1944) -> ()
                n636 = local write "tfalg"(1.0 ("tfalg")) -> ()
                n637 = local write "acq 2"(FALSE ("acq 2")) -> ()
                n638 = Wait (ms)(milliseconds to wait=u32 200) -> ()  [unwired: 1 out]
              }
            }
          }
        }
        n639 = case shown="False" w1846 {
          frame False {
            n640 = local read "zflag"() -> (→"zflag 2":dbl)
            n641 = local write "FLAG 4"(0.0 ("FLAG")) -> ()
            n642 = local write "yflag"(2.0 ("tflag")) -> ()
          }
          frame True {
            n643 = local write "zflag"(3.0 ("zflag")) -> ()
            n644 = local write "yflag"(1.0 ("tflag")) -> ()
          }
        }
        n645 = property on="STOP 3" class="Bool (strict)"() -> ("Visible"=w1848:bool)  [unwired: 2 in, 2 out]
        n646 = case shown="True" w1848 {
          tunnel: [FALSE ("Visible") TRUE ("Visible")] -> w1858
          frame False {
          }
          frame True {
          }
        }
        n647 = property on="RUN" class="Bool (strict)"("Visible"=w1858) -> ()  [unwired: 2 in, 2 out]
        n648 = property on="Save & Continue" class="Bool (strict)"() -> ("Visible"=w1861:bool)  [unwired: 2 in, 2 out]
        n649 = local read "RUN"() -> (w1842:bool)
        n650 = case shown="True" w1842 {
          frame False {
            n651 = local read "Rt 3"() -> (w1923:bool)
            n652 = case shown="True" w1923 {
              frame False {
              }
              frame True {
                n653 = local write "Json End Flg"(TRUE ("Upld AR 2")) -> ()
                n654 = local write "Rt 3"(FALSE ("Rt 3")) -> ()
              }
            }
            "Rt" <- TRUE ("Rt")
            "Rt 2" <- FALSE ("Rt")
          }
          frame True {
            n655 = local read "Rt"() -> (w1930:bool)
            n656 = case shown="True" w1930 {
              frame False {
              }
              frame True {
                w1931 = TRUE ("Upld AR 2")
                n657 = local write "Rt"(FALSE ("Rt")) -> ()
                n658 = local write "Upld AR"(w1931) -> ()
                n659 = local write "Json St Flg"(w1931) -> ()
              }
            }
            n660 = local write "Rt 2"(TRUE ("Rt 2")) -> ()
            "Rt 3" <- TRUE ("Rt 3")
          }
        }
        n661 = Not(x=w1861) -> (.not. x?=w1860:bool)
        n662 = case shown="True" w1842 {
          frame False {
            n663 = local write "run replace"(FALSE ("run replace")) -> ()
          }
          frame True {
            "run replace" <- TRUE ("run replace")
          }
        }
        n664 = And(x=w1860, y=w1848) -> (x .and. y?=w1857:bool)
        "Test Status 2" <- w1857
        n665 = case shown="True" w1857 {
          tunnel: w1806 -> [_ w1996]
          frame False {
            w1994 = 0.0 ("output")
            n666 = local write "PID-out"(w1994) -> ()
            n667 = local write "Heater Button"(FALSE ("Heater Button")) -> ()
            n668 = local write "Hz"(w1994) -> ()
          }
          frame True {
            n669 = case shown="False" w1996 {
              frame False {
                n670 = stacked-sequence {
                  frame #0 {
                    n671 = local write "RUN"(FALSE ("OK Button 2")) -> ()
                  }
                  frame #1 {
                    n672 = property on="RUN" class="Bool (strict)"("Visible"=FALSE) -> ()  [unwired: 2 in, 2 out]
                  }
                }
              }
              frame True {
              }
            }
            n673 = stacked-sequence {
              frame #0 {
                n674 = case shown="True" "RUN" {
                  tunnel: [w2023 w2031] -> w2000
                  frame False {
                    w2023 = 0.0
                    n675 = local write "Reinit PID"(TRUE) -> ()
                    n676 = property on="Stroke 2" class="DigNum (strict)"("Visible"=FALSE) -> ()  [unwired: 2 in, 2 out]
                    n677 = property on="Stroke" class="DigNum (strict)"("Visible"=TRUE) -> ()  [unwired: 2 in, 2 out]
                    n678 = local write "String 14"("Test will autostart once parameters reach the set value." ("String 14")) -> ()
                    n679 = local write "Old Pid Val"(w2023) -> ()
                  }
                  frame True {
                    n680 = local read "PID Ref"() -> (w2042:bool)
                    n681 = property on="STOP 2" class="Bool (strict)"("Disabled"=u8 2) -> ()  [unwired: 2 in, 2 out]
                    n682 = case shown="True" w2042 {
                      tunnel: [w2043 w2059] -> w2041
                      frame False {
                        n683 = local read "Old Pid Val"() -> (w2043:dbl)
                      }
                      frame True {
                        n684 = local read "Set Hz"() -> (w2052:dbl)
                        n685 = Add(x=w2052, y=-10.0 ("Offset")) -> (x+y=w2070:dbl)
                        n686 = local read "Frequency"() -> (w2063:dbl)
                        n687 = Add(x=w2052, y=-10.0) -> (x+y=w2062:dbl)
                        n688 = Add(x=w2052, y=10.0) -> (x+y=w2061:dbl)
                        n689 = Multiply(x=w2070, y=0.1 ("Gain")) -> (x*y=w2049:dbl)
                        n690 = Add(x=w2049, y=1.5) -> (x+y=w2047:dbl)
                        n691 = local read "SPEED OUT:"() -> (w2071:dbl)
                        n692 = In Range and Coerce(upper limit=w2061, x=w2063, lower limit=w2062) -> (coerced(x)=w2051:dbl)  [unwired: 1 out]
                        n693 = Multiply(x=w2047, y=w2071) -> (x*y=w2046:dbl)
                        n694 = Multiply(x=w2046, y=0.8) -> (x*y=w2045:dbl)
                        n695 = local read "Elapsed time"() -> (w2056:dbl)
                        n696 = Or(x="Reinit PID", y="Reinit PID") -> (x .or. y?=w2060:bool)
                        n697 = call-poly <vilib>:"PID.vi"("reinitialize? (F)"=w2060, "output range"=cluster{"output high":dbl, "output low":dbl} {"output high"=1.0, "output low"=-1.0}, "PID gains"=T4 {"proportional gain (Kc)"=0.0005, "integral time (Ti, min)"=0.001, "derivative time (Td, min)"=0.0} ("Motor PID"), "process variable"=w2051, "setpoint"=w2052) -> ("output"=w2050:dbl)  [unwired: 5 in, 1 out]
                        n698 = Greater?(x=w2056, y=0.05) -> (0:w2055:bool)
                        n699 = case shown="True" w2055 {
                          tunnel: w2050 -> [_ w2073]
                          tunnel: [0.0 ("output") w2073] -> w2053
                          frame False {
                          }
                          frame True {
                            n700 = local write "Reinit PID"(FALSE ("Reinit PID")) -> ()
                          }
                        }
                        n701 = Add(x=w2045, y=w2053) -> (x+y=w2058:dbl)
                        n702 = flat-sequence {
                          tunnel: [w2076] -> w2059
                          tunnel: w2058 -> [w2076]
                          frame #0 {
                            n703 = local write "PID Ref"(FALSE ("PID Ref")) -> ()
                          }
                        }
                      }
                    }
                    "Old Pid Val" <- w2041
                    n704 = local read "Set Hz"() -> (w2038:dbl)
                    n705 = local read "Freq"() -> (w2030:dbl)
                    n706 = call <vilib>:"Uniform White Noise Waveform.vi"() -> ("signal out"=w2037:waveform(dbl))  [unwired: 10 in, 1 out]
                    n707 = property on="RUN" class="Bool (strict)"("Visible"=TRUE) -> ()  [unwired: 2 in, 2 out]
                    n708 = Add(x=w2038, y=w2037) -> (x+y=w2036:waveform(dbl))
                    n709 = property on="Stroke 2" class="DigNum (strict)"("Visible"=TRUE) -> ()  [unwired: 2 in, 2 out]
                    n710 = property on="Stroke" class="DigNum (strict)"("Visible"=FALSE) -> ()  [unwired: 2 in, 2 out]
                    n711 = Multiply(x=w2036, y=ext 0.1) -> (x*y=w2032:waveform(ext))
                    n712 = Multiply(x=w2030, y=0.9) -> (x*y=w2033:dbl)
                    n713 = local write "String 14"(" Running....." ("String 14")) -> ()
                    n714 = Add(x=w2032, y=w2033) -> (x+y=w2031:waveform(ext))
                  }
                }
                n715 = Not(x="Engage") -> (.not. x?=w2004:bool)
                n716 = call "Elapsed Time"("Time Target (s)"="Countdown", "Reset"=w2004) -> ("Elapsed Time (s)"=w2009:dbl, "Time has Elapsed"=w2007:bool)  [unwired: 10 in, 6 out]
                "Countdown 2" <- w2009
                n717 = Subtract(x=w2009, y=2.0) -> (x-y=w2012:dbl)
                n718 = Less?(x=w2012, y="Countdown") -> (x < y?=w2010:bool)
                n719 = And(x=w2010, y=w2007) -> (x .and. y?=w2006:bool)
                n720 = case shown="True" w2006 {
                  frame False {
                  }
                  frame True {
                    n721 = local read "Humidity"() -> (→"Rh Before":dbl)
                    n722 = local write "RUN"(TRUE ("RUN")) -> ()
                    n723 = local write "Engage"(FALSE ("Engage")) -> ()
                    n724 = property on="gRh" class="WFChart (strict)"("History Data"=dbl[] []) -> ()  [unwired: 2 in, 2 out]
                  }
                }
                n725 = local read "clk"() -> (w2017:dbl)
                n726 = local read "Save"() -> (w2013:bool)
                n727 = Equal?(x=w2017, y=0.0) -> (x = y?=w2014:bool)
                n728 = And(x=w2014, y=w2013) -> (x .and. y?=w2015:bool)
                n729 = case shown="True" w2015 {
                  frame False {
                  }
                  frame True {
                    n730 = Get Date/Time In Seconds() -> (seconds since 1Jan1904=w2079:timestamp)
                    n731 = To Double Precision Float(number=w2079) -> (double precision float=w2077:dbl)
                    n732 = local write "act save time"(w2077) -> ()
                    n733 = local write "acq timer"(w2077) -> ()
                    n734 = local write "clk"(10.0 ("clk")) -> ()
                  }
                }
                n735 = local read "Test \nStatus"() -> (w2002:bool)
                n736 = Select(t=w2000, s=w2002, f=0.0) -> (s? t:f=w2001:dbl)
                n737 = local write "Freq"(w2001) -> ()
                n738 = local write "Hz"(w2001) -> ()
              }
              frame #1 {
                w2102 = 1000000.0 ("x")
                # "Elapsed time\ncof\nstroke\nAir temp\nTemp\nHumidity"
                # "acq timer\n\nact save time"
                # "convert to microseconds"
                n739 = local read "COUNT"() -> (w2085:i32)
                n740 = Greater Or Equal?(x=w2085, y=250) -> (x >= y?=w2084:bool)
                n741 = case shown="True" w2084 {
                  frame False {
                    n742 = local read "COUNT"() -> (w2106:i32)
                    n743 = Increment(x=w2106) -> (x+1=w2107:i32)
                    n744 = local write "COUNT"(w2107) -> ()
                  }
                  frame True {
                    n745 = local write "COUNT"(0 ("COUNT")) -> ()
                  }
                }
                n746 = local read "Samplingtime 2"() -> (w2083:dbl)
                n747 = local read "act save time"() -> (w2100:dbl)
                n748 = Get Date/Time In Seconds() -> (seconds since 1Jan1904=w2105:timestamp)
                n749 = To Double Precision Float(number=w2105) -> (double precision float=w2094:dbl)
                n750 = local read "acq timer"() -> (w2104:dbl)
                n751 = Add(x=w2100, y=w2083) -> (x+y=w2099:dbl)
                n752 = Greater Or Equal?(x=w2094, y=w2099) -> (x >= y?=w2082:bool)
                n753 = Subtract(x=w2094, y=w2104) -> (x-y=w2096:dbl)
                n754 = local read "Rate"() -> (w2098:dbl)
                n755 = Divide(x=w2102, y=w2098) -> (x/y=w2103:dbl)
                n756 = Divide(x=w2103, y=w2102) -> (x/y=w2101:dbl)
                n757 = local read "Save"() -> (w2097:bool)
                n758 = And(x=w2082, y=w2097) -> (x .and. y?=w2095:bool)
